vi "end.vi"(8 "error in (no error)":errorcluster, 11 "Communication Channel in":refnum<class "Communication Channel.lvclass">) -> (0 "error out":errorcluster, 3 "Communication Channel out":refnum<class "Communication Channel.lvclass">)   [LabVIEW 2018, in "Communication Channel.lvclass"]
uses:
  Communication Channel.lvclass
  Socket/Socket.lvclass
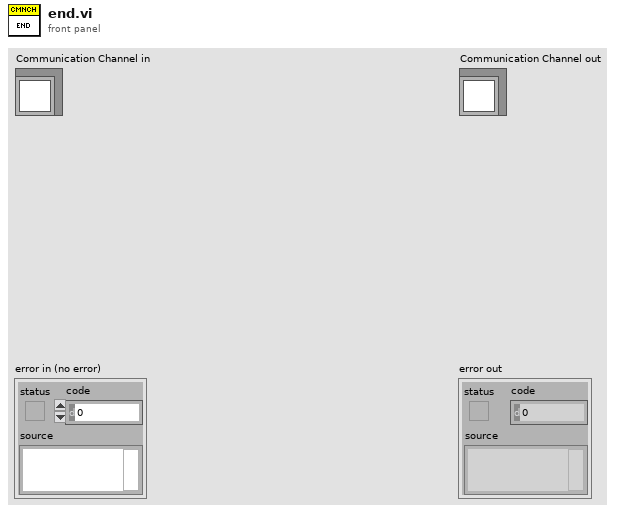
[diagram p1: front panel]
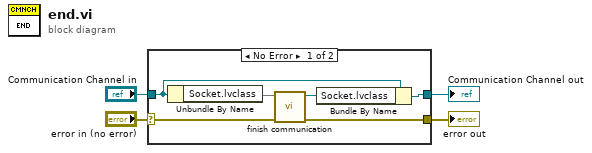
[diagram p0: block diagram]
diagram:
  n1 = case shown="No Error" "error in (no error)" {
    selector: "error in (no error)" -> [w10 w12]
    tunnel: [w9 w12] -> w3
    tunnel: [w6 w11] -> w1
    tunnel: "Communication Channel in" -> [w7 w11]
    frame No Error {
      n2 = Unbundle By Name(w7) -> ("Socket.lvclass"=w8)
      n3 = call-dynamic "finish communication.vi"("error in (no error)"=w10, "Socket in"=w8) -> ("error out"=w9:errorcluster, "Socket out"=w5:refnum<class "Socket.lvclass">)  [unwired: 8 in]
      n4 = Bundle By Name(cluster=w7, "Socket.lvclass"=w5) -> (w6:refnum<class "Communication Channel.lvclass">)
    }
    frame Error {
    }
  }
  "error out" <- w3
  "Communication Channel out" <- w1
